vi "Database.Cache.Changeover.vi"(7 "Idx":i32, 8 "error in":errorcluster, 11 "Ref":string) -> (0 "error out":errorcluster, 2 "TS out":T1 {"TS"."TP"."value" format="%#.3f"; "TS"."TV"."minimum" format="%#.3f"; "TS"."TV"."maximum" format="%#.3f"})   [LabVIEW 2016]
doc: "Write test results (measurement values) to proda database\n\nWabco 2017 All right reserved\nAuthor: maciej.szupienko@wabco-auto.com"
uses:
  Cache/Cache.TestSteps.Fglb.TestData.ctl
  ProdaNG/Controls/ProdaNG.Process.ctl
  ProdaNG/Controls/ProdaNG.ProcessStep.ctl
  ProdaNG/Controls/ProdaNG.ProcessStepParam.ctl
  ProdaNG/Controls/ProdaNG.TestStep.ctl
  ProdaNG/Controls/ProdaNG.TestValue.ctl
  ProdaNG/Controls/ProdaNG.TestStepParam.ctl
  ProdaNG/Controls/ProdaNG.Unit.ctl
  Tools/EventLog/EventLog.EventSource.ctl
  Cache/Cache.Status.Fglb.Action.ctl
  Cache/Cache.TestSteps.Fglb.Action.ctl
  Cache/Cache.TestSteps.Fglb.ResultData.ctl
  ProdaNG/Controls/ProdaNG.ProcessResult.ctl
  ProdaNG/Controls/ProdaNG.ProcessStepResult.ctl
  ProdaNG/Controls/ProdaNG.TestStepResult.ctl
  ProdaNG/Controls/ProdaNG.TestValueResult.ctl
  Tools/Translator/Translator.Message.ctl
  Tools/EventLog/EventLog.New(single).vi
  Database.Global.vi
  Global/ApplicationGlobal.vi
  Tools/EventLog/EventLog.Buffer.vi
  Tools/EventLog/EventLog.File.ReadWrite.vi
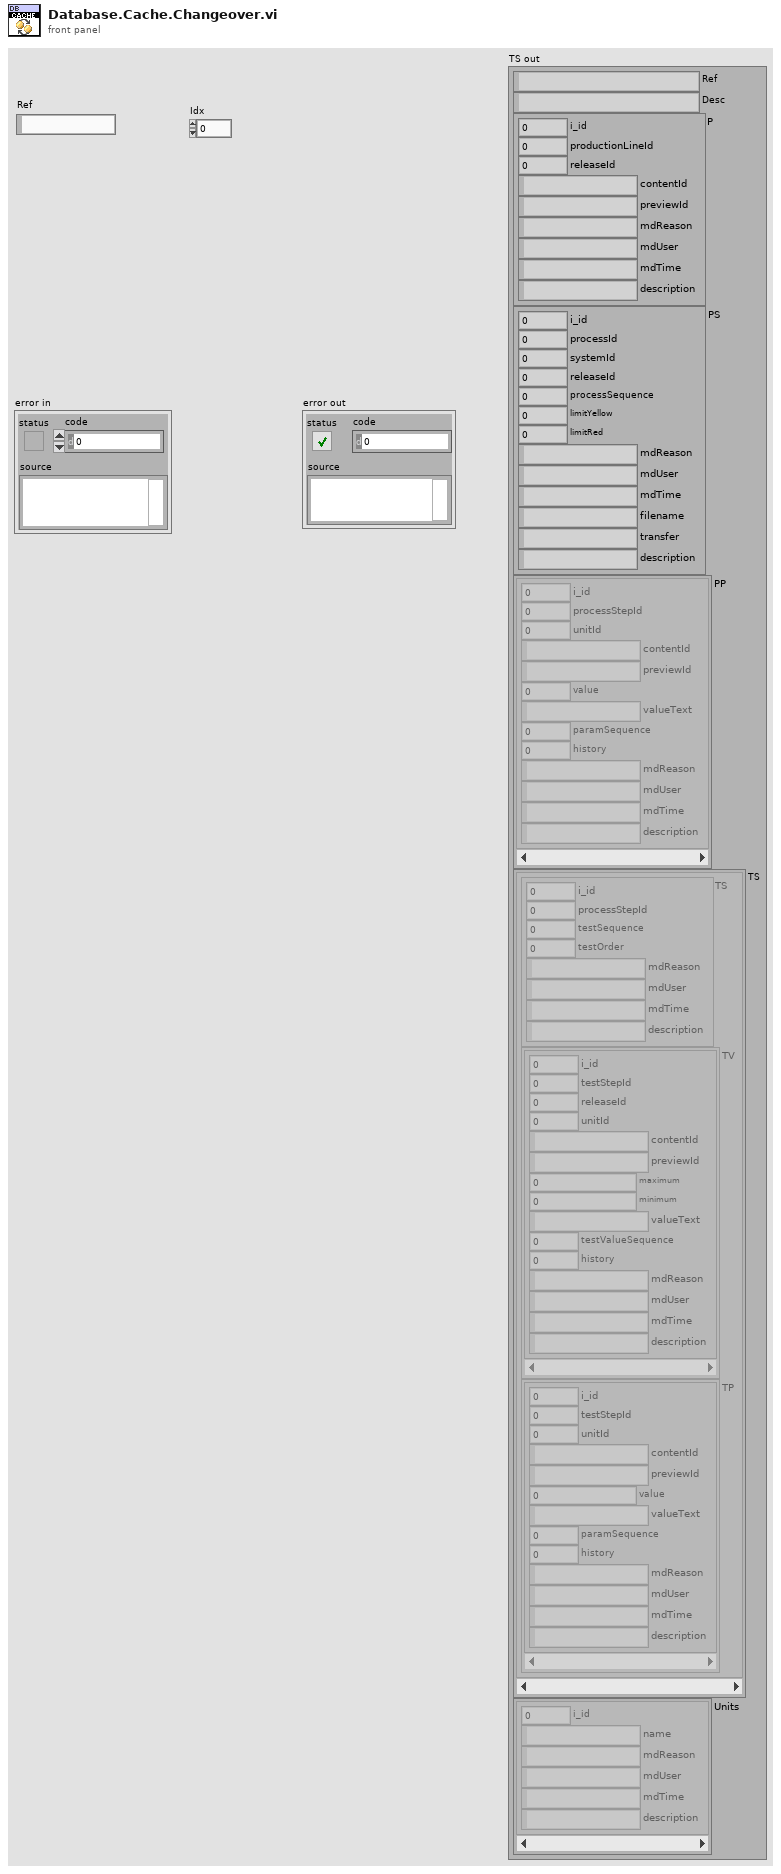
[diagram p1: front panel]
types:
  T1 = typedef "Cache.TestSteps.Fglb.TestData.ctl" = cluster{"Ref":string, "Desc":string, "P":T2, "PS":T3, "PP":T4[], "TS":cluster{"TS":T5, "TV":T6[], "TP":T7[]}[], "Units":T8[]}
  T2 = typedef "ProdaNG.Process.ctl" = cluster{"i_id":i32, "productionLineId":i32, "releaseId":i32, "contentId":string, "previewId":string, "mdReason":string, "mdUser":string, "mdTime":string, "description":string}
  T3 = typedef "ProdaNG.ProcessStep.ctl" = cluster{"i_id":i32, "processId":i32, "systemId":i32, "releaseId":i32, "processSequence":i32, "limitYellow":dbl, "limitRed":dbl, "mdReason":string, "mdUser":string, "mdTime":string, "filename":string, "transfer":string, "description":string}
  T4 = typedef "ProdaNG.ProcessStepParam.ctl" = cluster{"i_id":i32, "processStepId":i32, "unitId":i32, "contentId":string, "previewId":string, "value":dbl, "valueText":string, "paramSequence":i32, "history":i32, "mdReason":string, "mdUser":string, "mdTime":string, "description":string}
  T5 = typedef "ProdaNG.TestStep.ctl" = cluster{"i_id":i32, "processStepId":i32, "testSequence":i32, "testOrder":i32, "mdReason":string, "mdUser":string, "mdTime":string, "description":string}
  T6 = typedef "ProdaNG.TestValue.ctl" = cluster{"i_id":i32, "testStepId":i32, "releaseId":i32, "unitId":i32, "contentId":string, "previewId":string, "maximum":dbl, "minimum":dbl, "valueText":string, "testValueSequence":i32, "history":i32, "mdReason":string, "mdUser":string, "mdTime":string, "description":string}
  T7 = typedef "ProdaNG.TestStepParam.ctl" = cluster{"i_id":i32, "testStepId":i32, "unitId":i32, "contentId":string, "previewId":string, "value":dbl, "valueText":string, "paramSequence":i32, "history":i32, "mdReason":string, "mdUser":string, "mdTime":string, "description":string}
  T8 = typedef "ProdaNG.Unit.ctl" = cluster{"i_id":i32, "name":string, "mdReason":string, "mdUser":string, "mdTime":string, "description":string}
  T9 = typedef "Cache.Status.Fglb.Action.ctl" = enum16{"init", "Changeover", "CheckStatus", "NewData", "get"}
  T10 = typedef "EventLog.EventSource.ctl" = enum16{"All", "Gui", "Cache", "PLC1", "PLC2", "PLC3", "DB", "DB01", "DB02", "DB03", "DB04", "DB05", "DB06", "DB07", "DB08", "DB09", "DB10", "DB11", "DB12", "DB13", "DB14", "DB15", "DB16"}
  T11 = typedef "Translator.Message.ctl" = enum16{"-", "Event confirmed", "Log out", "Log in", "Shutdown", "Cancel", "Start", "Continue", "Stop", "On", "Off", "OK", "NOK", "NOK %s", "This", "Prev", "Home", "Work", "In progress...", "Missing", "Empty", "Hardware failure", "Initial", "Error %d >> %s", "Error %d >> %s >> %s", "Starting %s", "Quitting %s", "Configured", "Initializing", "Quitting", "Loading", "Running %s", "Stopped", "Summary", "Do you want to continue?", "Do you want to exit?", "Log out?", "System", "All", "IDLE", "Translating...%s", "Not found", "Alarm %s", "Run", "Skip", "Abort", "Repeat", "Please wait...", "Database disconnected", "Login to database successful", "Login to database failed: %d; %s", "Get process step data for %s", "Changeover off", "Changeover into %s", "Product %s | %s found in cache with status %d at previous station", "Product %s | %s found in database with status %d at previous station", "Product %s | %s not found in cache at previous station", "Product %s | %s not found in database at previous station", "Product %s | %s found in cache with status %d at this station (%d repetion)", "Product %s | %s found in database with status %d at this station (%d repetition)", "Product %s | %s not found in cache at this station", "Product %s | %s not found in database at this station", "Product %s | %s found in cache for component %s | %s", "Product %s | %s found in database for component %s | %s", "Product not found in cache for component %s | %s", "Product not found in database for component %s | %s", "Product %s | %s connected with component %s | %s (cache)", "Product %s | %s connected with component %s | %s (database)", "New data for %s | %s (cache)", "New data for %s | %s (database)", "File %s moved (cache)", "File %s deleted (cache)", "Msg %d >> %s", "PLC LifeBit Failure", "Reconnecting DB", "Reconnecting PLC", "Free disk space is below 1GB - contact technician", "Unable to check product status", "Product %s SN %s checked in DB", "Unable To check status from station %s"}
  T12 = typedef "Cache.TestSteps.Fglb.ResultData.ctl" = cluster{"File":path, "Ref":string, "Serial":string, "Pr":T13, "PSr":T14, "TSr":cluster{"TSr":T15, "TVr":T16[]}[]}
  T13 = typedef "ProdaNG.ProcessResult.ctl" = cluster{"c_id":string, "productId":string, "processId":i32, "statusId":i32, "startTime":string, "endTime":string}
  T14 = typedef "ProdaNG.ProcessStepResult.ctl" = cluster{"c_id":string, "processResultId":string, "processStepId":i32, "statusId":i32, "operatorId":i32, "startTime":string, "endTime":string}
  T15 = typedef "ProdaNG.TestStepResult.ctl" = cluster{"c_id":string, "processStepResultId":string, "testStepId":i32, "statusId":i32}
  T16 = typedef "ProdaNG.TestValueResult.ctl" = cluster{"c_id":string, "testStepResultId":string, "testValueId":i32, "result":dbl, "statusId":i32, "contentId":string}
  T17 = typedef "Cache.TestSteps.Fglb.Action.ctl" = enum16{"init", "add", "get"}
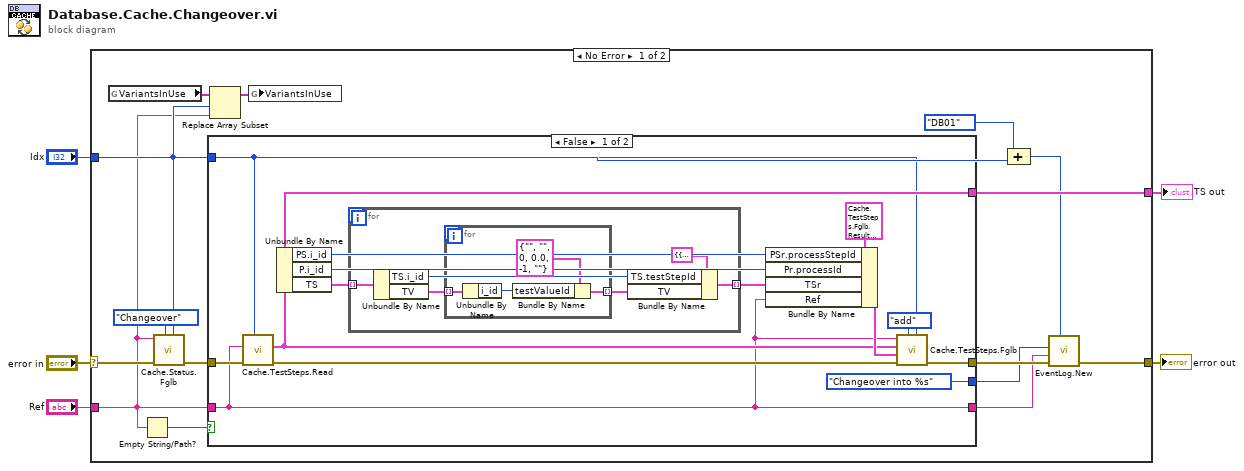
[diagram p0: block diagram]
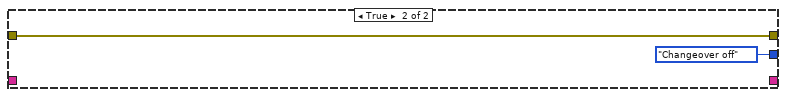
[diagram p2: hidden frame]
diagram:
  n1 = case shown="No Error" "error in" {
    selector: "error in" -> [w12 w47]
    tunnel: [w18 w47] -> w5
    tunnel: "Idx" -> [w8 _]
    tunnel: "Ref" -> [w7 _]
    tunnel: [w20 _] -> w1
    frame No Error {
      n2 = global read "Database.Global.vi" "VariantsInUse"() -> (w9:string[])
      n3 = Empty String/Path?(string/path=w7) -> (empty?=w19:bool)
      n4 = call "Cache.Status.Fglb.vi"("SystemIdx"=w8, "Action (get)"=Cache.Status.Fglb.Action."Changeover", "error in (no error)"=w12, "Changeover"=w7) -> ("error out"=w11:errorcluster)  [unwired: 6 in, 1 out]
      n5 = case shown="False" w19 {
        tunnel: w11 -> [w26 w46]
        tunnel: [w25 w46] -> w17
        tunnel: [w24 _] -> w20
        tunnel: w8 -> [w23 _]
        tunnel: w7 -> [w21 _]
        tunnel: [Translator.Message."Changeover into %s" ("Message (-)") Translator.Message."Changeover off" ("Message (-)")] -> w16
        tunnel: [w21 _] -> w15
        frame False {
          n6 = call "Cache.TestSteps.Read.vi"("Idx"=w23, "error in (no error)"=w26, "Ref"=w21) -> ("error out"=w31:errorcluster, "TS in"=w24:T1)  [unwired: 7 in]
          n7 = Unbundle By Name(w24) -> ("PS.i_id"=w28:i32, "P.i_id"=w29:i32, "TS"=w34:cluster{"TS":T5, "TV":T6[], "TP":T7[]}[])
          n8 = for {
            tunnel: [w37] -> w27 mode=indexing
            tunnel: w34 -> [w36] mode=indexing
            n9 = Unbundle By Name(w36) -> ("TS.i_id"=w39:i32, "TV"=w35:T6[])
            n10 = for {
              tunnel: w35 -> [w44] mode=indexing
              tunnel: [w41] -> w40 mode=indexing
              n11 = Unbundle By Name(w44) -> ("i_id"=w43:i32)
              n12 = Bundle By Name(cluster=T16 {"c_id"="", "testStepResultId"="", "testValueId"=0, "result"=0.0, "statusId"=-1, "contentId"=""} ("TV"), "testValueId"=w43) -> (w41:T16)
            }
            n13 = Bundle By Name(cluster=cluster{"TS":T15, "TV":T16[]} {"TS"={"c_id"="", "processStepResultId"="", "testStepId"=0, "statusId"=-1}, "TV"=[]} ("Cluster"), "TS.testStepId"=w39, "TV"=w40) -> (w37:cluster{"TS":T15, "TV":T16[]})
          }
          n14 = Bundle By Name(cluster=T12 {"File"=path "", "Ref"="", "Serial"="", "Pr"={"c_id"="", "productId"="", "processId"=0, "statusId"=0, "startTime"="", "endTime"=""}, "PSr"={"c_id"="", "processResultId"="", "processStepId"=0, "statusId"=0, "operatorId"=0, "startTime"="", "endTime"=""}, "TSr"=[]} ("Result in"), "PSr.processStepId"=w28, "Pr.processId"=w29, "TSr"=w27, "Ref"=w21) -> (w32:T12)
          n15 = call "Cache.TestSteps.Fglb.vi"("SystemIdx"=w23, "Action (get)"=Cache.TestSteps.Fglb.Action."add", "error in (no error)"=w31, "Result in"=w32, "Test in"=w24, "Variant"=w21) -> ("error out"=w25:errorcluster)  [unwired: 2 in, 3 out]
        }
        frame True {
        }
      }
      n16 = Replace Array Subset(array=w9, new element=w7, index=w8) -> (w6:string[])
      n17 = global write "Database.Global.vi" "VariantsInUse"(w6) -> ()
      n18 = Compound Arithmetic op=ADD(EventLog.EventSource."DB01" ("Source (All)"), w8) -> (w13:i32)
      n19 = call-poly "EventLog.New.vi"("Source (All)"=w13, "error in (no error)"=w17, "Arg"=w15, "Message (-)"=w16) -> ("error out"=w18:errorcluster)  [unwired: 6 in, 1 out]
    }
    frame Error {
    }
  }
  "error out" <- w5
  "TS out" <- w1
